vi "Main_CLIWrapper.vi"(11 "Inputs":string[](array[string])) -> (2 "Output/Failure":string, 3 "CLI Process Return Code":i32)   [LabVIEW 2019]
uses:
  <vilib>/Utility/error.llb/DialogType.ctl
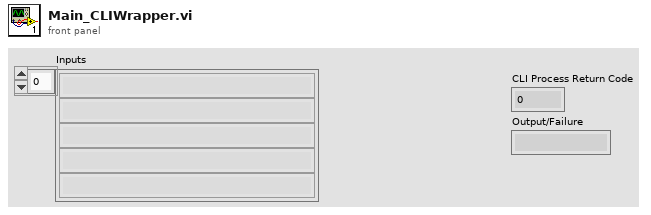
[diagram p1: front panel]
types:
  T1 = typedef "DialogType.ctl" = u16
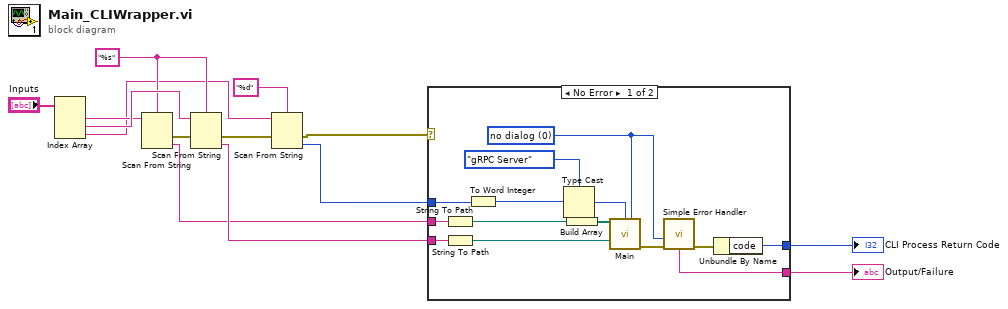
[diagram p0: block diagram]
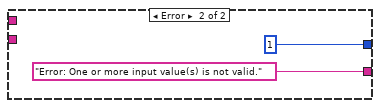
[diagram p2: hidden frame]
diagram:
  w12 = "%s" ("format string")
  n1 = Index Array "Index Array"(array="Inputs") -> (element #1=w10:string, element #2=w13:string, element #3=w8:string)  [unwired: 3 in]
  n2 = Scan From String(format string=w12, input string=w10) -> (error out=w11:errorcluster, output 1=w3:string)  [unwired: 3 in, 2 out]
  n3 = Scan From String(format string=w12, input string=w13, error in=w11) -> (error out=w7:errorcluster, output 1=w4:string)  [unwired: 2 in, 2 out]
  n4 = Scan From String(format string="%d", input string=w8, error in=w7) -> (error out=w1:errorcluster, output 1=w2:i32)  [unwired: 2 in, 2 out]
  n5 = case shown="No Error" w1 {
    tunnel: [w23 1] -> w6
    tunnel: [w20 "Error: One or more input value(s) is not valid."] -> w5
    tunnel: w4 -> [w25 _]
    tunnel: w3 -> [w28 _]
    tunnel: w2 -> [w16 _]
    frame No Error {
      w19 = T1 0 items=["no dialog", "OK message", "continue or stop message", "OK message + warnings", "continue/stop + warnings"] ("type of dialog (OK msg:1)")
      n6 = String To Path(string=w28) -> (path=w27:path)
      n7 = String To Path(string=w25) -> (path=w24:path)
      n8 = To Word Integer(number=w16) -> (16bit integer=w15:i16)
      n9 = Type Cast(type=enum16{"gRPC Server", "gRPC Client", "Both"}."gRPC Server" ("Generate"), x=w15) -> (*(type *) &x=w17:enum16{"gRPC Server", "gRPC Client", "Both"})
      n10 = Build Array(w27) -> (w26:path[])
      n11 = call <vilib>:"Main.vi"("Proto File Path"=w26, "Generate Server or Client?"=w17, "type of dialog (OK msg:1)"=w19, "Target Project"=w24) -> ("error out"=w22:errorcluster)  [unwired: 11 in]
      n12 = call <vilib>:"Simple Error Handler.vi"("type of dialog (OK msg:1)"=w19, "error in (no error)"=w22) -> ("error out"=w21:errorcluster, "message"=w20:string)  [unwired: 3 in, 3 out]
      n13 = Unbundle By Name(w21) -> ("code"=w23:i32)
    }
    frame Error {
    }
  }
  "CLI Process Return Code" <- w6
  "Output/Failure" <- w5
